vi "CalcDiv_Multiple_From_Folder.vi"() -> ()   [LabVIEW 2017]
uses:
  <vilib>/Utility/file.llb/Write Delimited Spreadsheet (DBL).vi
panel:
  out "Divergence":dbl[](array[numeric])
  out "Angle":dbl[](array[numeric])
  in  "Calc Divergence":bool
  out "Width":cluster{i32[], dbl[]}[](graph)
  out "Centroid":cluster{i32[], dbl[]}[](graph)
  out "Slow Axis Array":T1(array[cluster])
  out "Fast Axis Array":T1(array[cluster])
  in  "Pixel size, um":dbl=5.5 format="%#_13g"
  in  "Rotate, deg":dbl format="%#_13g"
  out "Index":i32[](array[numeric])
  in  "pattern":string="*.bmp"
  in  "AOI":cluster{"AOI h, px":dbl, "AOI w, px":dbl}
  in  "Folder Path":path
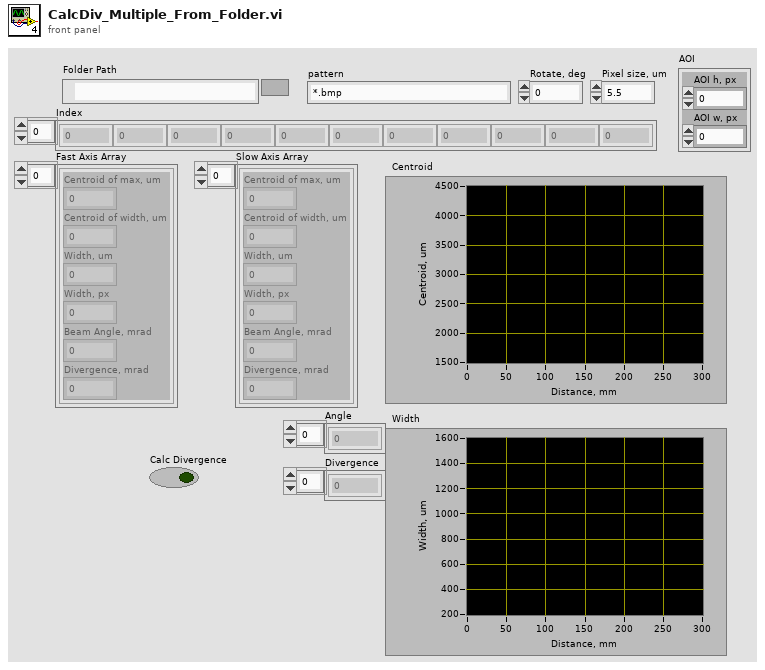
[diagram p1: front panel]
types:
  T1 = cluster{"Centroid of max, um":dbl, "Centroid of width, um":dbl, "Width, um":dbl, "Width, px":i32, "Beam Angle, mrad":dbl, "Divergence, mrad":dbl}[]
  T2 = cluster{"Centroid of max, um":dbl, "Centroid of width, um":dbl, "Width, um":dbl, "Width, px":i32, "Beam Angle, mrad":dbl, "Divergence, mrad":dbl}
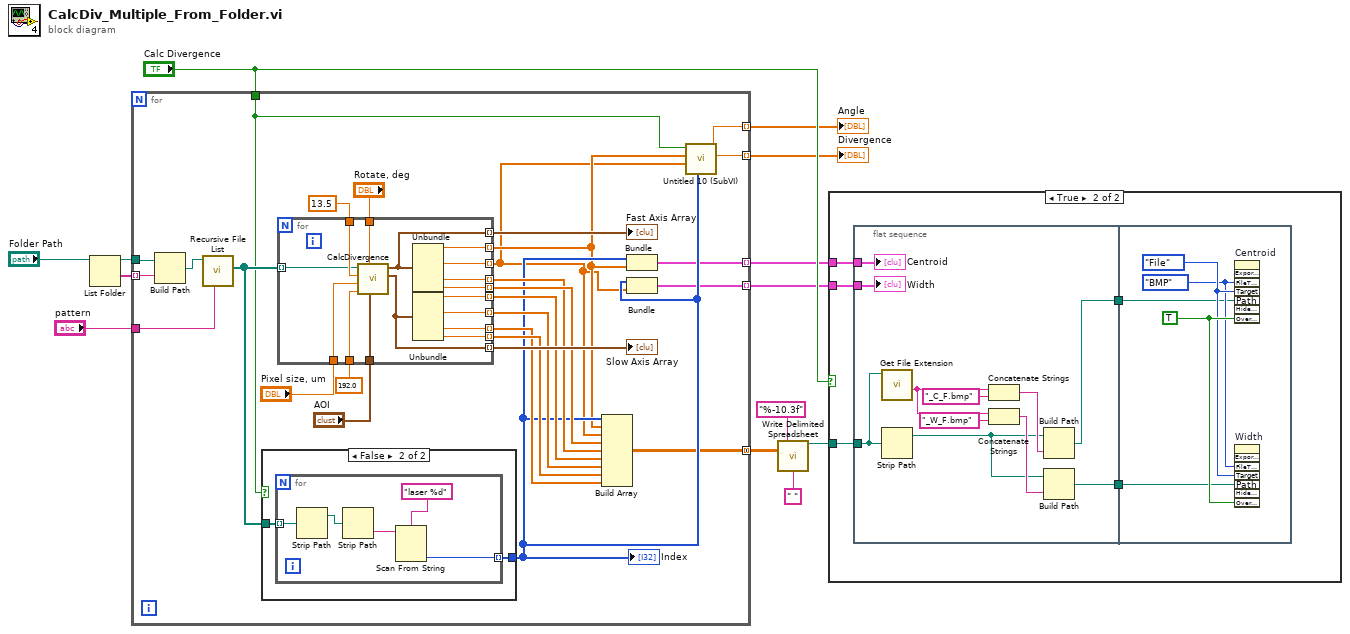
[diagram p0: block diagram]
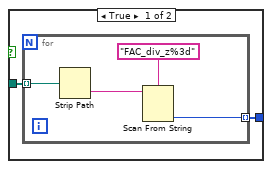
[diagram p2: hidden frame]
diagram:
  n1 = List Folder(path="Folder Path") -> (path out=w3:path, folder names=w2:string[])  [unwired: 3 in, 2 out]
  n2 = for {
    tunnel: "Calc Divergence" -> [w23]
    tunnel: [w22] -> w12 mode=indexing
    tunnel: [w21] -> w11 mode=indexing
    tunnel: [w20] -> w10 mode=indexing
    tunnel: [w19] -> w9 mode=indexing
    tunnel: [w18] -> w7 mode=concatenating
    tunnel: w3 -> [w17]
    tunnel: w2 -> [w16] mode=indexing
    tunnel: "pattern" -> [w14]
    n3 = Build Path(base path=w17, name or relative path=w16) -> (appended path=w15:path)
    n4 = call <vilib>:"Recursive File List.vi"("pattern"=w14, "Folder Path"=w15) -> ("All Files in Dir"=w35:path[])  [unwired: 5 in, 4 out]
    n5 = case shown="False" w23 {
      tunnel: w35 -> [w42 w48]
      tunnel: [w41 w47] -> w26
      frame True {
        n6 = for {
          tunnel: w42 -> [w44] mode=indexing
          tunnel: [w43] -> w41 mode=indexing
          n7 = Strip Path(path=w44) -> (name=w46:string)  [unwired: 1 out]
          n8 = Scan From String(format string="FAC_div_z%3d", input string=w46) -> (output 1=w43:i32)  [unwired: 3 in, 3 out]
        }
      }
      frame False {
        n9 = for {
          tunnel: w48 -> [w52] mode=indexing
          tunnel: [w51] -> w47 mode=indexing
          n10 = Strip Path(path=w52) -> (stripped path=w50:path)  [unwired: 1 out]
          n11 = Strip Path(path=w50) -> (name=w49:string)  [unwired: 1 out]
          n12 = Scan From String(format string="laser %d", input string=w49) -> (output 1=w51:i32)  [unwired: 3 in, 3 out]
        }
      }
    }
    "Index" <- w26
    n13 = for {
      tunnel: w35 -> [w64] mode=indexing
      tunnel: "AOI" -> [w69]
      tunnel: 192.0 ("Focus, mm") -> [w68]
      tunnel: "Pixel size, um" -> [w67]
      tunnel: 13.5 ("Threshold, %") -> [w66]
      tunnel: "Rotate, deg" -> [w65]
      tunnel: [w63] -> w27 mode=indexing
      tunnel: [w62] -> w34 mode=indexing
      tunnel: [w61] -> w25 mode=indexing
      tunnel: [w60] -> w24 mode=indexing
      tunnel: [w59] -> w33 mode=indexing
      tunnel: [w58] -> w32 mode=indexing
      tunnel: [w57] -> w31 mode=indexing
      tunnel: [w56] -> w30 mode=indexing
      tunnel: [w55] -> w29 mode=indexing
      tunnel: [w54] -> w28 mode=indexing
      n14 = call "CalcDivergence.vi"("AOI"=w69, "Rotate, deg"=w65, "Focus, mm"=w68, "Pixel size, um"=w67, "Threshold, %"=w66, "path to file"=w64) -> ("Slow Axis"=w62:T2, "Fast Axis"=w63:T2)  [unwired: 4 in]
      n15 = Unbundle(w63) -> ("Centroid of max, um"=w61:dbl, "Width, um"=w60:dbl, "Beam Angle, mrad"=w58:dbl, "Divergence, mrad"=w59:dbl)  [unwired: 2 out]
      n16 = Unbundle(w62) -> ("Centroid of max, um"=w57:dbl, "Width, um"=w56:dbl, "Beam Angle, mrad"=w54:dbl, "Divergence, mrad"=w55:dbl)  [unwired: 2 out]
    }
    "Fast Axis Array" <- w27
    "Slow Axis Array" <- w34
    n17 = Build Array(w26, w25, w24, w33, w32, w31, w30, w29, w28) -> (w18:dbl[][])
    n18 = Bundle(w26, w25) -> (w22:cluster{i32[], dbl[]})  [unwired: 1 in]
    n19 = Bundle(w26, w24) -> (w21:cluster{i32[], dbl[]})  [unwired: 1 in]
    n20 = call "Untitled 10 (SubVI).vi"("Array 3"=w26, "Array"=w24, "Array 2"=w25, "Calc Divergence"=w23) -> ("mean"=w19:dbl, "mean 2"=w20:dbl)  [unwired: 6 in]
  }
  "Angle" <- w10
  "Divergence" <- w9
  n21 = call-poly <vilib>:"Write Delimited Spreadsheet.vi"("format (%.3f)"="%-10.3f", "2D data"=w7, "delimiter (\\t)"=" " ("delimiter (\\t)")) -> ("new file path (Not A Path if cancelled)"=w5:path)  [unwired: 11 in, 1 out]
  n22 = case shown="True" "Calc Divergence" {
    tunnel: w12 -> [_ w72]
    tunnel: w11 -> [_ w71]
    tunnel: w5 -> [_ w70]
    frame False {
    }
    frame True {
      n23 = flat-sequence {
        tunnel: w72 -> [w85]
        tunnel: w71 -> [w84]
        tunnel: w70 -> [w83]
        tunnel: [w77] -> w74
        tunnel: [w76] -> w73
        tunnel: w74 -> [w87]
        tunnel: w73 -> [w86]
        frame #0 {
          n24 = call <vilib>:"Get File Extension.vi"("file"=w83) -> ("filename without extension"=w80:string)  [unwired: 6 in, 4 out]
          n25 = Strip Path(path=w83) -> (stripped path=w75:path)  [unwired: 1 out]
          n26 = Concatenate Strings(w80, "_C_F.bmp" ("string")) -> (w79:string)
          n27 = Concatenate Strings(w80, "_W_F.bmp" ("string")) -> (w78:string)
          n28 = Build Path(base path=w75, name or relative path=w79) -> (appended path=w76:path)
          n29 = Build Path(base path=w75, name or relative path=w78) -> (appended path=w77:path)
          "Centroid" <- w85
          "Width" <- w84
        }
        frame #1 {
          w89 = enum32{"File", "Clipboard"}."File" ("Target")
          w90 = TRUE ("Always Overwrite")
          w88 = enum32{"BMP", "EPS", "EMF", "PICT"}."BMP" ("File Type")
          n30 = invoke on="Centroid" class="XYGraph (strict)" method="Export Image"("FileType"=w88, "Target"=w89, "Path"=w86, "Overwrite"=w90) -> ()  [unwired: 4 in, 8 out]
          n31 = invoke on="Width" class="XYGraph (strict)" method="Export Image"("FileType"=w88, "Target"=w89, "Path"=w87, "Overwrite"=w90) -> ()  [unwired: 4 in, 8 out]
        }
      }
    }
  }
